vi "GetFontsOSes__FD__LCR.vi"(8 "error in (no error)":errorcluster) -> (0 "error out":errorcluster, 3 "SystemFonts":string[](array[string]))   [LabVIEW 2011]
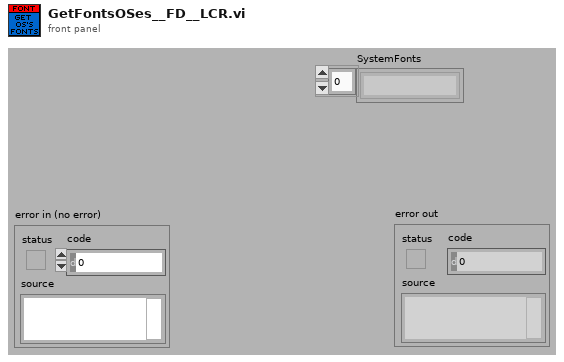
[diagram p1: front panel]
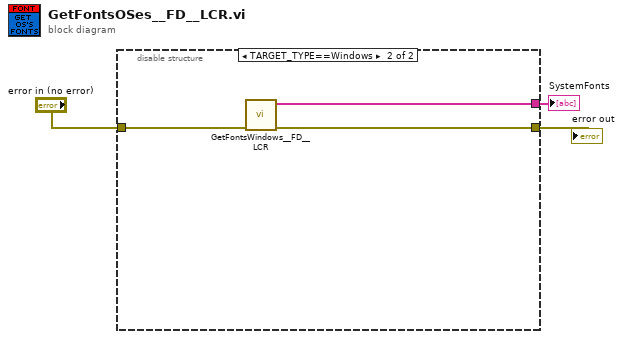
[diagram p0: block diagram]
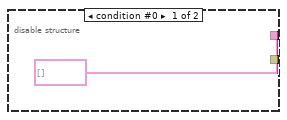
[diagram p2: hidden frame]
diagram:
  n1 = disable-structure shown="TARGET_TYPE==Windows" {
    disable-tunnel: [string[] [] w7] -> w1
    disable-tunnel: "error in (no error)" -> [_ w6]
    disable-tunnel: [_ w5] -> w2
    frame condition #0 {
    }
    frame condition #1 (active) {
      n2 = call "GetFontsWindows__FD__LCR.vi"("error in (no error)"=w6) -> ("error out"=w5:errorcluster, "Fonts"=w7:string[])  [unwired: 9 in]
    }
  }
  "error out" <- w2
  "SystemFonts" <- w1
